vi "RPOPLPUSH.vi"(0 "refnum in":refnum<vi>, 5 "Source":string, 7 "Destination":string, 11 "error in":errorcluster) -> (4 "refnum out":refnum<vi>, 6 "Data":T1, 15 "error out":errorcluster)   [LabVIEW 2020]
uses:
  SubVIs/Controls/redis-data.ctl
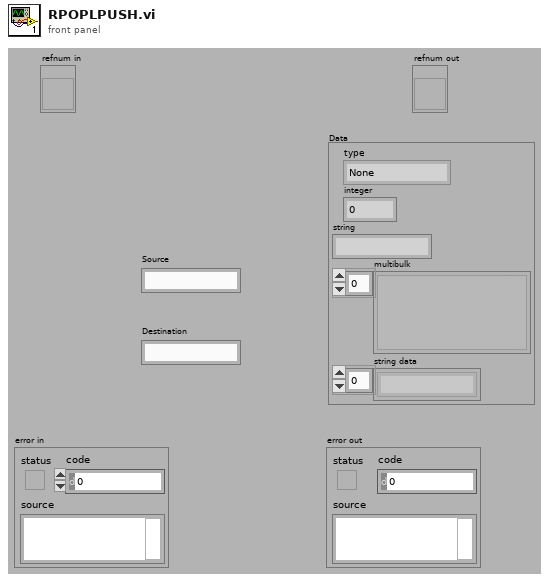
[diagram p1: front panel]
types:
  T1 = typedef "redis-data.ctl" = cluster{"type":enum16{"None", "Error", "Status", "Nil", "Integer", "String", "Multibulk"}, "integer":i64, "string":string, "multibulk":variant[], "string data":string[]}
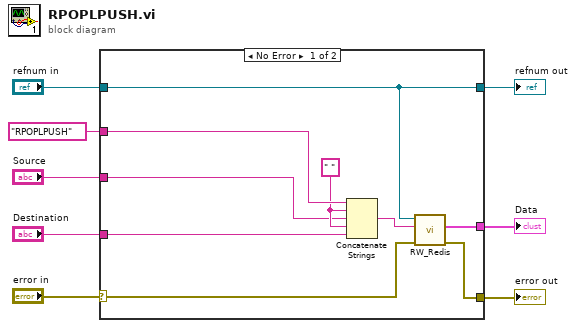
[diagram p0: block diagram]
diagram:
  n1 = case shown="No Error" "error in" {
    selector: "error in" -> [w16 w19]
    tunnel: "RPOPLPUSH" -> [w13 _]
    tunnel: "refnum in" -> [w9 w18]
    tunnel: [w15 w19] -> w6
    tunnel: [w14 _] -> w2
    tunnel: "Source" -> [w11 _]
    tunnel: "Destination" -> [w10 _]
    tunnel: [w9 w18] -> w1
    frame No Error {
      w12 = " "
      n2 = Concatenate Strings(w13, w12, w11, w12, w10) -> (w17:string)
      n3 = call "RW_Redis.vi"("error in"=w16, "command"=w17, "refnum"=w9) -> ("error out"=w15:errorcluster, "Data"=w14:T1)  [unwired: 7 in]
    }
    frame Error {
    }
  }
  "error out" <- w6
  "refnum out" <- w1
  "Data" <- w2
